vi "Destroy User Event.vi"(8 "error in (no error)":errorcluster caption="エラー入力（エラーなし）", 11 "User Event":refnum<user-event> caption="ユーザイベント") -> (0 "error out":errorcluster caption="エラー出力")   [LabVIEW 2014]
doc: "エラーを受信してもユーザイベントを破棄します。"
uses:
  Ctl/Event Cluster.ctl
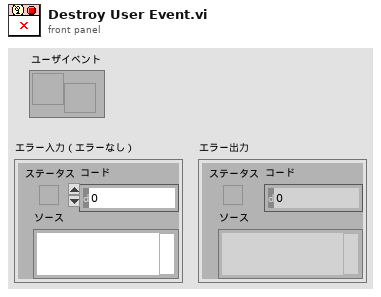
[diagram p1: front panel]
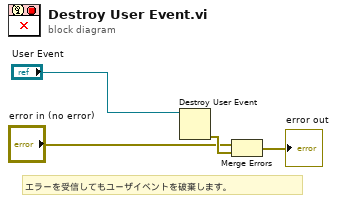
[diagram p0: block diagram]
diagram:
  # "エラーを受信してもユーザイベントを破棄します。"
  n1 = Destroy User Event(user event="User Event") -> (error out=w3:errorcluster)  [unwired: 1 in]
  n2 = Merge Errors("error in (no error)", w3) -> (→"error out":errorcluster)
